vi "ParseVI.vi"(11 "VIPath":string) -> (2 "数组":string[][](array[string]), 3 "VIInfo":cluster{"Name":string, "Terminals":T1[]})   [LabVIEW 2018]
uses:
  Ctr/TerminalInfo.ctl
  Ctr/VIInfo.ctl
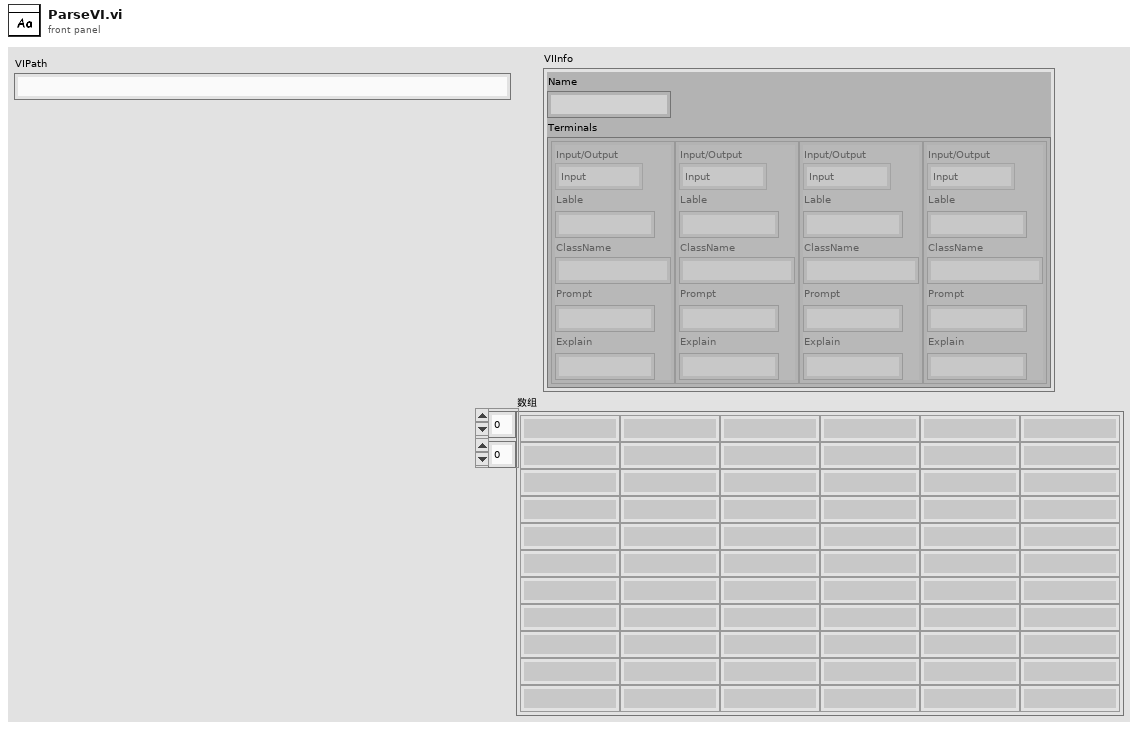
[diagram p1: front panel]
types:
  T1 = typedef "TerminalInfo.ctl" = cluster{"Input/Output":T2, "Lable":string, "ClassName":string, "Prompt":string, "Explain":string}
  T2 = typedef "IsIndicator" = enum16{"Input", "Output"}
  T3 = typedef "VIInfo.ctl" = cluster{"Name":string, "Terminals":T1[]}
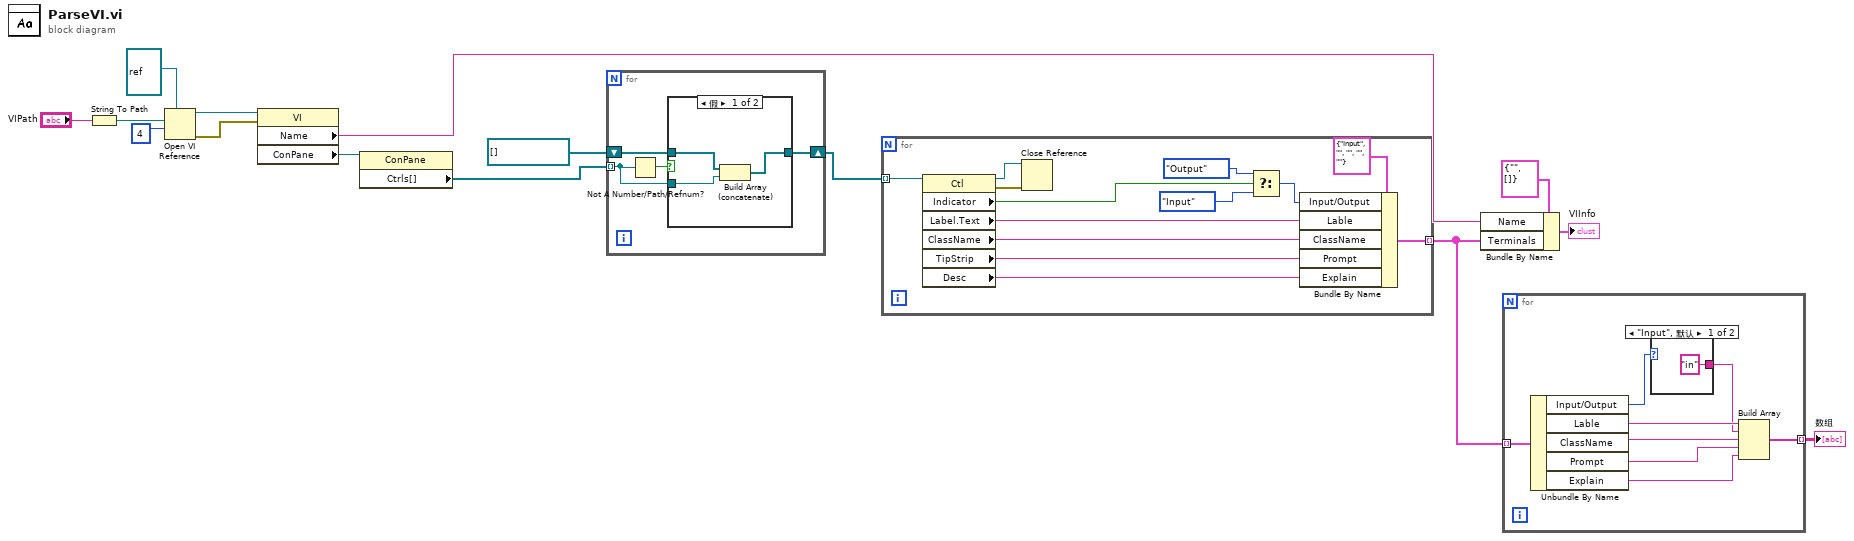
[diagram p0: block diagram]
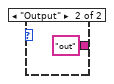
[diagram p2: hidden frame]
diagram:
  n1 = String To Path(string="VIPath") -> (path=w8:path)
  n2 = Open VI Reference(type specifier VI Refnum (for type only)=refnum<vi> refnum ("类型说明符VI引用句柄（仅用于类型）"), vi path=w8, options=4 ("选项")) -> (vi reference=w10:refnum<vi>, error out=w9:errorcluster)  [unwired: 3 in]
  n3 = property class="VI"(reference=w10, error in=w9) -> ("Name"=w15:string, "ConPane"=w7:refnum<vi>)  [unwired: 2 out]
  n4 = property class="ConPane"(reference=w7) -> ("Ctrls[]"=w5:refnum<vi>[])  [unwired: 1 in, 2 out]
  n5 = for {
    tunnel: w5 -> [w18] mode=indexing
    shift-right: [w17] -> w3
    shift-left: refnum<vi>[] [] -> [w16]
    n6 = Not A Number/Path/Refnum?(number/path/refnum=w18) -> (NaN/Path/Refnum?=w19:bool)
    n7 = case shown="假" w19 {
      tunnel: w18 -> [w22 _]
      tunnel: [w21 w23] -> w17
      tunnel: w16 -> [w20 w23]
      frame False {
        n8 = Build Array (concatenate)(w20, w22) -> (w21:refnum<vi>[])
      }
      frame True {
      }
    }
  }
  n9 = for {
    tunnel: w3 -> [w36] mode=indexing
    tunnel: [w26] -> w2 mode=indexing
    n10 = property class="Ctl"(reference=w36) -> (reference out=w25:refnum<vi>, error out=w24:errorcluster, "Indicator"=w32:bool, "Label.Text"=w33:string, "ClassName"=w34:string, "TipStrip"=w28:string, "Desc"=w27:string)  [unwired: 1 in]
    n11 = Close Reference(reference=w25, error in (no error)=w24) -> ()  [unwired: 1 out]
    n12 = Select(t=IsIndicator."Output" ("Input/Output"), s=w32, f=IsIndicator."Input" ("Input/Output")) -> (s? t:f=w29:T2)
    n13 = Bundle By Name(cluster=T1 {"Input/Output"=enum."Input", "Lable"="", "ClassName"="", "Prompt"="", "Explain"=""} ("NewCluster"), "Input/Output"=w29, "Lable"=w33, "ClassName"=w34, "Prompt"=w28, "Explain"=w27) -> (w26:T1)
  }
  n14 = Bundle By Name(cluster=T3 {"Name"="", "Terminals"=[]} ("输入簇"), "Name"=w15, "Terminals"=w2) -> (→"VIInfo":T3)
  n15 = for {
    tunnel: w2 -> [w44] mode=indexing
    tunnel: [w37] -> w1 mode=indexing
    n16 = Unbundle By Name(w44) -> ("Input/Output"=w39:T2, "Lable"=w43:string, "ClassName"=w40:string, "Prompt"=w41:string, "Explain"=w42:string)
    n17 = case shown="\"Input\", 默认" w39 {
      tunnel: ["in" "out"] -> w38
      frame "Input", Default {
      }
      frame "Output" {
      }
    }
    n18 = Build Array(w43, w38, w40, w41, w42) -> (w37:string[])
  }
  "数组" <- w1
